vi "GUI_map_image_parser.vi"(0 "color":u32(colorbox), 1 "Thickness":u8, 4 "zoom#":dbl=70.0, 5 "Image Src":T2, 6 "Ctl Refnum":refnum<vi>, 7 "Image Dst":T2, 8 "Image options":T1, 9 "size":cluster{"xhair size":dbl, "xhair size 2":dbl}={"xhair size"=20.0, "xhair size 2"=20.0} {"xhair size 2" min=0.0 max=0.0; "xhair size" min=0.0 max=0.0}, 10 "target y":dbl=0.001 caption="Y" min=0.0 max=2000.0, 11 "target x":dbl=0.001 caption="X" min=0.0 max=2000.0) -> (2 "ms timer out":u32, 3 "Img out":T2(plugin-control) caption="M1 Cam")   [LabVIEW 2020]
uses:
  <vilib>/vision/Image Controls.llb/IMAQ Image.ctl
  General GUIs/shared/Image GUI options.ctl
  General GUIs/Device GUIs/GUI_Cameras/Controls/Crosshair type def.ctl
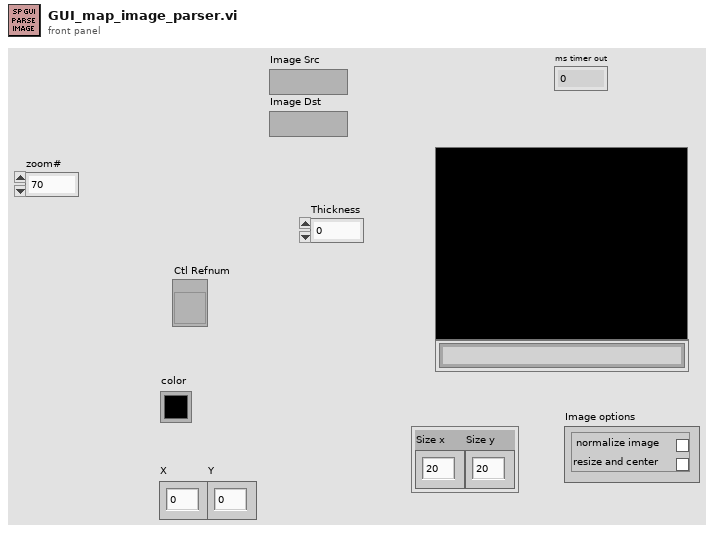
[diagram p1: front panel]
types:
  T1 = typedef "Image GUI options.ctl" = cluster{"normalize image":bool, "resize and center":bool}
  T2 = typedef "IMAQ Image.ctl" = refnum<image>
  T3 = typedef "Crosshair type def.ctl" = cluster{"Draw":bool, "Target":cluster{"x":dbl, "y":dbl}, "Size":cluster{"x":dbl, "y":dbl}, "Angle":dbl, "Color":u32, "Thickness":u8, "CrosshairLabel":string}
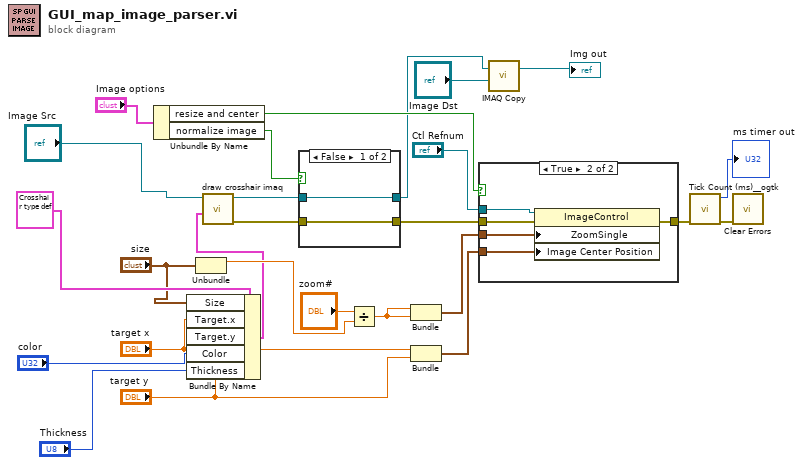
[diagram p0: block diagram]
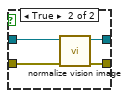
[diagram p2: hidden frame]
diagram:
  n1 = Unbundle By Name("Image options") -> ("resize and center"=w15:bool, "normalize image"=w11:bool)
  n2 = Bundle By Name(cluster=T3 {"Draw"=TRUE, "Target"={"x"=25.0, "y"=25.0}, "Size"={"x"=25.0, "y"=25.0}, "Angle"=0.0, "Color"=8322834, "Thickness"=1, "CrosshairLabel"=""} ("Crosshair"), "Size"="size", "Target.x"="target x", "Target.y"="target y", "Color"="color", "Thickness"="Thickness") -> (w3:T3)
  n3 = Unbundle("size") -> ("xhair size"=w12:dbl)  [unwired: 1 out]
  n4 = call "draw crosshair imaq.vi"("Crosshair"=w3, "image in"="Image Src") -> ("error out"=w13:errorcluster, "image out"=w26:T2)  [unwired: 8 in]
  n5 = case shown="False" w11 {
    tunnel: w26 -> [w28 w32]
    tunnel: [w28 w31] -> w8
    tunnel: [w27 w30] -> w20
    tunnel: w13 -> [w27 w29]
    frame False {
    }
    frame True {
      n6 = call "normalize vision image.vi"("error in (no error)"=w29, "Refnum in"=w32) -> ("error out"=w30:errorcluster, "Refnum out"=w31:T2)  [unwired: 7 in, 1 out]
    }
  }
  n7 = Divide(x="zoom#", y=w12) -> (x/y=w23:dbl)
  n8 = Bundle(w23, w23) -> (w25:cluster{dbl, dbl})  [unwired: 1 in]
  n9 = Bundle("target x"="target x", "target y"="target y") -> (w22:cluster{"target x":dbl, "target y":dbl})  [unwired: 1 in]
  n10 = case shown="True" w15 {
    tunnel: w25 -> [_ w38]
    tunnel: w22 -> [_ w37]
    tunnel: [w33 w36] -> w21
    tunnel: w20 -> [w33 w35]
    tunnel: "Ctl Refnum" -> [_ w34]
    frame False {
    }
    frame True {
      n11 = property on="Property Node" class="ImageControl"(reference=w34, error in=w35, "ZoomSingle"=w38, "Image Center Position"=w37) -> (error out=w36:errorcluster)  [unwired: 1 out]
    }
  }
  n12 = call "IMAQ Copy"("Image Dst"="Image Dst", "Image Src"=w8) -> ("Image Dst Out"=→"Img out":T2)  [unwired: 4 in, 1 out]
  n13 = call <userlib>:"Tick Count (ms)__ogtk.vi"("error in (no error)"=w21) -> ("error out"=w14:errorcluster, "millisecond timer value"=→"ms timer out":u32)  [unwired: 9 in]
  n14 = call <vilib>:"Clear Errors.vi"("error in (no error)"=w14) -> ()  [unwired: 5 in, 2 out]
